vi "Serial_Kart.vi"(4 "string to write":string="*IDN?", 5 "error in (no error)":errorcluster, 7 "VISA resource name":refnum<visa-resource-name>) -> (0 "read string":string, 1 "error out":errorcluster)   [LabVIEW 2011]
doc: "The Advanced Serial Read and Write example performs a Serial Port Read, a Serial Port Write, or a combination of these actions while setting some advanced serial features like buffer size, termination characters, and XON/XOFF flow control. The user selects the actions (read or write) on the front panel. If both are selected, the VI will write the data first, read the data and then close the VISA session that is opened to the port. \n\nThe parameters set for the serial port must match the parameters of the connected instrument or device. In this example, the bytes to read parameter specifies the number of bytes that the serial port reads. If there were more bytes at the port than the number specified in bytes to read, those bytes would not be read. Also, if you specify to read more bytes than the number of bytes actually read, you might receive a timeout error message.\n\nINSTRUCTIONS:\n1) Select the serial resource and configuration parameters (baud rate, data bits, parity, stop bits, flow control).\n2) Termination character can be enabled and set. Also, set the required input buffer size prior to running the example.\n3) Select the operations to be performed. \n4) Connect the serial port to your device. If no device is available, perform a loopback test by doing one of the following. Short pins 2 and 3 on a RS-232 cable or short pin 4 to pin 8 and pin 5 to pin 9 on a RS-485/422 cable. \n5) Run the VI to see the data read. (The \"read string\" will match the \"string to write\" if a loopback test was performed.)\n\nThis example exposes several advanced features that you may need for your application. Not all applications need all the features shown in this example. The input buffer size is likely an important setting that you want to control in your application. This example expands upon the flow control option for XON and XOFF, allowing the user to choose those control characters. The timeout parameter has been brought to the front panel so a user can specify the time period the VISA Read will wait for the number of bytes to read before timing out. Also, the user has several controls for the termination character, which is discussed later.\n\nNote that you can press the write and read buttons and change the bytes to read parameters on the fly, while the example is running. However, you must stop the example to change the other configuration parameters after the example has started running, and then run again.\n\nSet the I/O buffer size slightly higher the amount of data you expect to receive. This is very important for applications that don't use flow control, as you may lose characters if the receive buffer overflows.\n\nSetting the timeout period ensures that the operation returns with a timeout error if the operation cannot be performed in the specified time period. \n\nSome devices require a termination character in order to identify the end of command strings. Some devices send a termination character to signify the end of data to be read. \n\nThis example shows how you can end the Read operation once a termination character is detected in the buffer and/or append a termination character at the end of the Write data. To enable the Read to end on a termination character, use the VISA Configure Serial Port or use the VISA Properties Serial End Mode for Reads, Termination Character Enable, and Termination Character. To end the Write with a termination character, use the VISA Properties Serial End Mode for Writes, the Send End Enable, and Termination Character. In this example, the same termination character is used for both the Read and the Write. You can specify two different characters for your application, if desired.\n\nYour application may require specific characters for the XON/XOFF Flow Control. You can specify these characters with the VISA Properties Flow Control XOFF Character and Flow Control XON Character. Note that if the standard XON and XOFF characters are used, then decimal 17 and 19 are unavailable for data values. Remember that using flow control and setting an adequate buffer size allow you to prevent buffer overflows."
panel:
  out "actual bytes read":u32
  out "bytes written":u32
  # "On Windows/Linux, consider using the Instrument Driver Finder (Help>>Find Instrument Drivers) to search for an instrument driver for your instrument."
  # "Select the serial resource and the operations to be performed.  If all are selected, the VI will write the data first, read data and then close the VISA session that is opened to the port.  This VI will wait until the specified number of bytes is received at the port, until the timeout period is met, or until a termination character is received.  The default termination character in this example is the Line Feed ( ASCII 0xA, '\\n' ).  Also, set the required input buffer size prior to running the example.\nNote: The example loops until the STOP button is pressed."
  # "For additional information select File >> VI Properties >> Documentation"
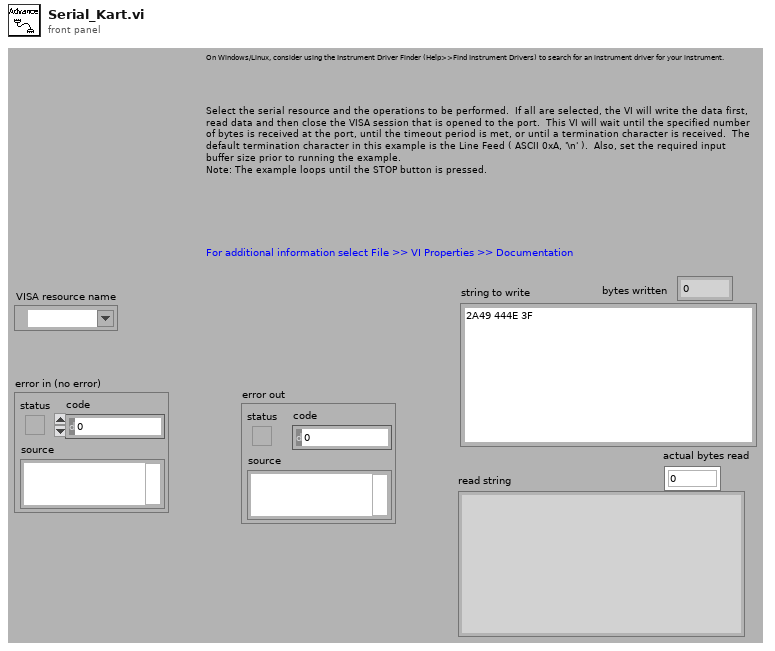
[diagram p1: front panel]
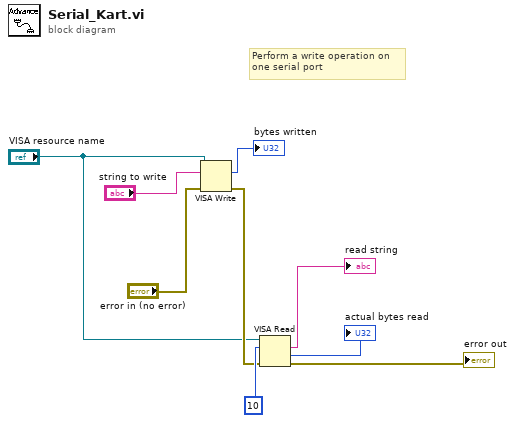
[diagram p0: block diagram]
diagram:
  # "Perform a write operation on one serial port"
  n1 = VISA Write(VISA resource name="VISA resource name", write buffer="string to write", error in (no error)="error in (no error)") -> (return count=→"bytes written":u32, error out=w4:errorcluster)  [unwired: 1 out]
  n2 = VISA Read(VISA resource name="VISA resource name", byte count=u32 10, error in (no error)=w4) -> (read buffer=→"read string":string, return count=→"actual bytes read":u32, error out=→"error out":errorcluster)  [unwired: 1 out]
